vi "Test in Loop.vi"() -> ()   [LabVIEW 2020]
uses:
  99_Reference/LVMQTT-master/Controls/Connection_Return_Codes.ctl
  99_Reference/LVMQTT-master/Controls/QoS.ctl
  99_Reference/LVMQTT-master/Controls/User_Info.ctl
  99_Reference/LVMQTT-master/Controls/Connect_Flags.ctl
  99_Reference/LVMQTT-master/Controls/DUP_Flag.ctl
  99_Reference/LVMQTT-master/Controls/Retain_Flag.ctl
  <vilib>/NI/AMC/Read Termination Message.vi
  <vilib>/NI/AMC/Create Single Message.vi
  <vilib>/NI/AMC/Update Message Routing Info.vi
  <vilib>/NI/AMC/Globals.vi
  <vilib>/NI/AMC/Send Message.vi
  <vilib>/ErrorRing/Error Ring.xnode
  99_Reference/LVMQTT-master/MQTT_Functions.lvlib
  <vilib>/NI/AMC/AMC.lvlib
  <userlib>/_OpenG.lib/time/time.llb/openg_time.lvlib
panel:
  in  "Read":bool
  in  "CMD_0":bool
  in  "Test Connect":bool
  out "Connection Status":T1
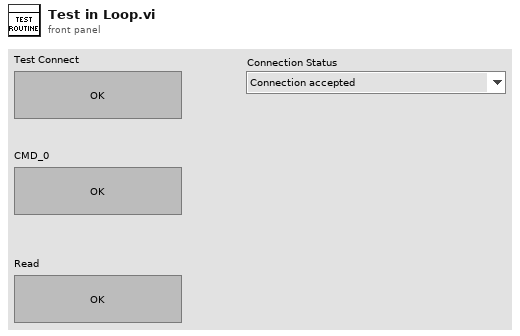
[diagram p1: front panel]
types:
  T1 = typedef "MQTT_Functions.lvlib/Connection_Return_Codes.ctl" = enum16{"Connection accepted", "Connection refused: unacceptable protocol version", "Connection refused: identifier rejected", "Connection refused: Server unavailable", "Connection refused: bad user name or password", "Connection refused: not authorized"}
  T2 = typedef "AMC.lvlib/Message Queue.ctl" = refnum<queue>
  T3 = typedef "MQTT_Functions.lvlib/QoS.ctl" = enum8{"At most once", "At least once", "Exactly once", "Reserved"}
  T4 = typedef "MQTT_Functions.lvlib/Retain_Flag.ctl" = bool
  T5 = typedef "MQTT_Functions.lvlib/DUP_Flag.ctl" = bool
  T6 = cluster{"Hostname":string, "Mac(From)":string, "IP":string, "ConnID":refnum<k5>}
  T7 = cluster{"QoS":T3, "DUP":T5, "Retain":T4, "Keep Alive (sec)":u16}
  T8 = typedef "MQTT_Functions.lvlib/Connect_Flags.ctl" = cluster{"user name":bool, "password":bool, "will retain":bool, "will flag":bool, "clean session":bool, "reserved":bool, "will QoS":T3}
  T9 = typedef "MQTT_Functions.lvlib/User_Info.ctl" = cluster{"User Name":string, "Password":string}
  T10 = cluster{"User Info":T9, "Client ID":string, "MQTT Broker":cluster{"address (IP)":string, "port":u16}, "Connection Status":T1, "Connect Flags":T8, "Connect Meta":cluster{"QoS":T3, "DUP":T5, "Retain":T4, "Keep Alive (sec)":u16}, "MainInfo":cluster{"Hostname":string, "Mac(From)":string, "IP":string, "ConnID":refnum<k5>}, "Channel":string, "tickCount":u32, "tickTarget":u32, "Message ID":u16, "Subscription Info Array":cluster{"Topic":string, "QoS":T3}[]}
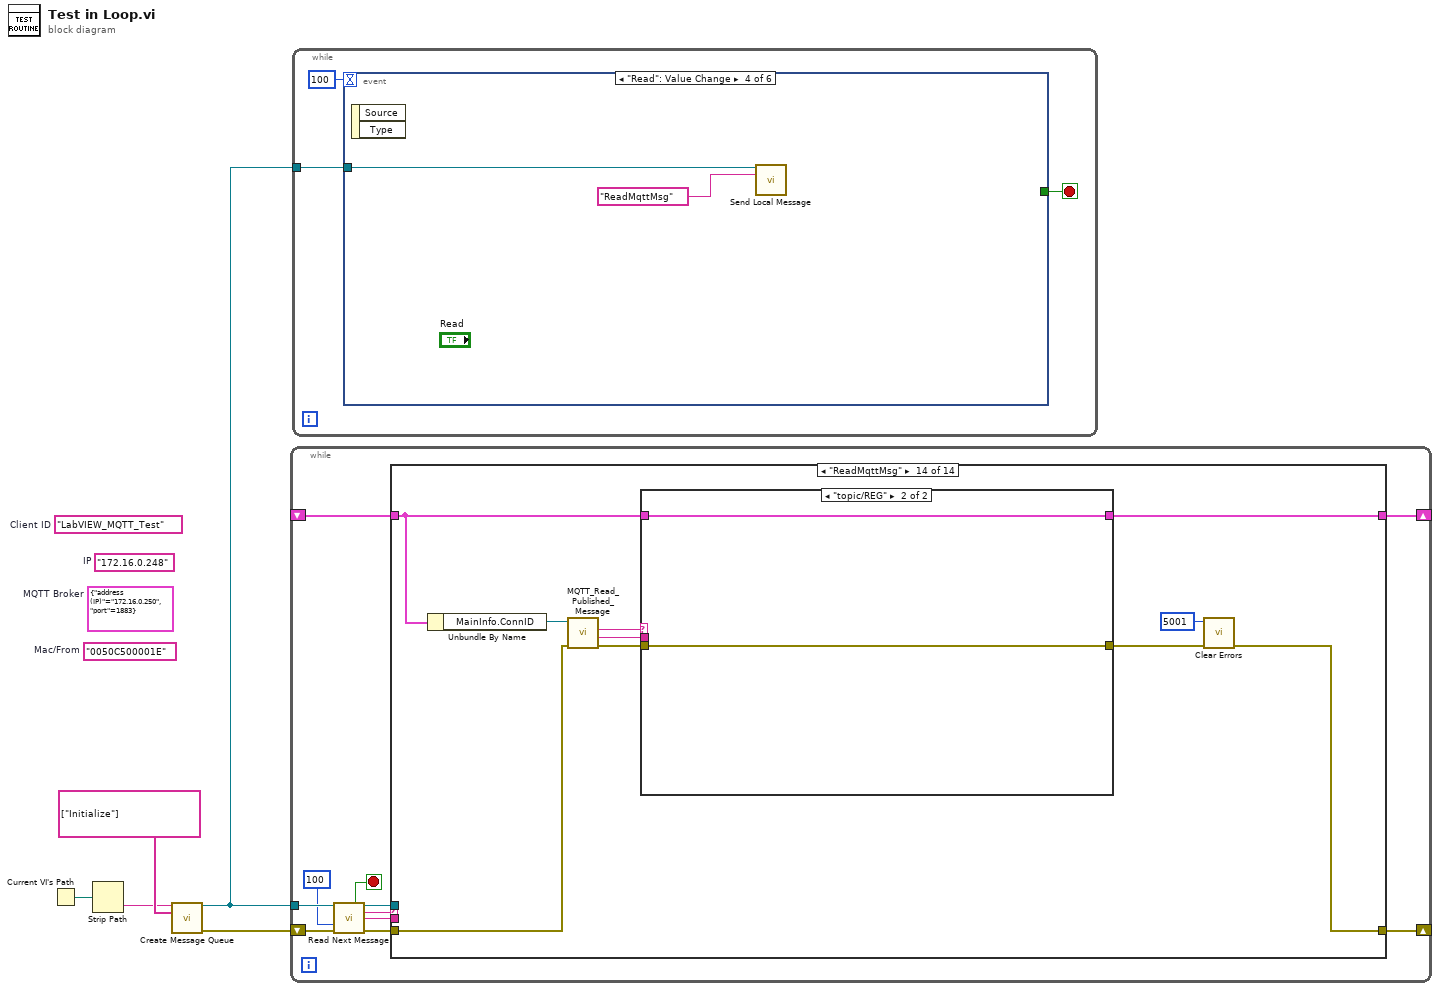
[diagram p0: block diagram]
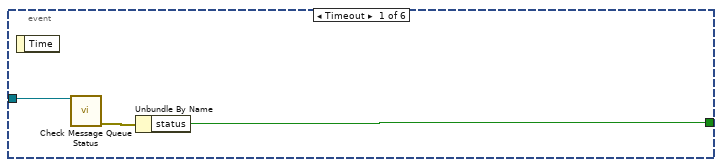
[diagram p2: hidden frame]
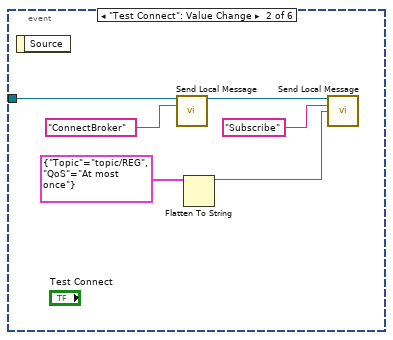
[diagram p3: hidden frame]
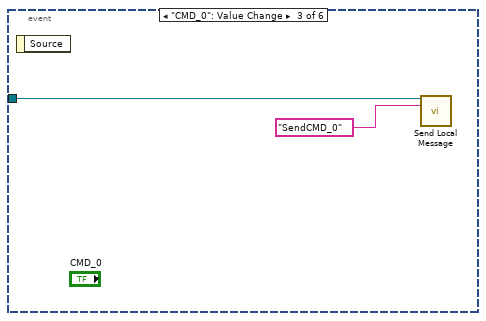
[diagram p4: hidden frame]
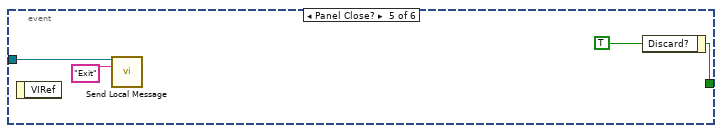
[diagram p5: hidden frame]
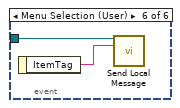
[diagram p6: hidden frame]
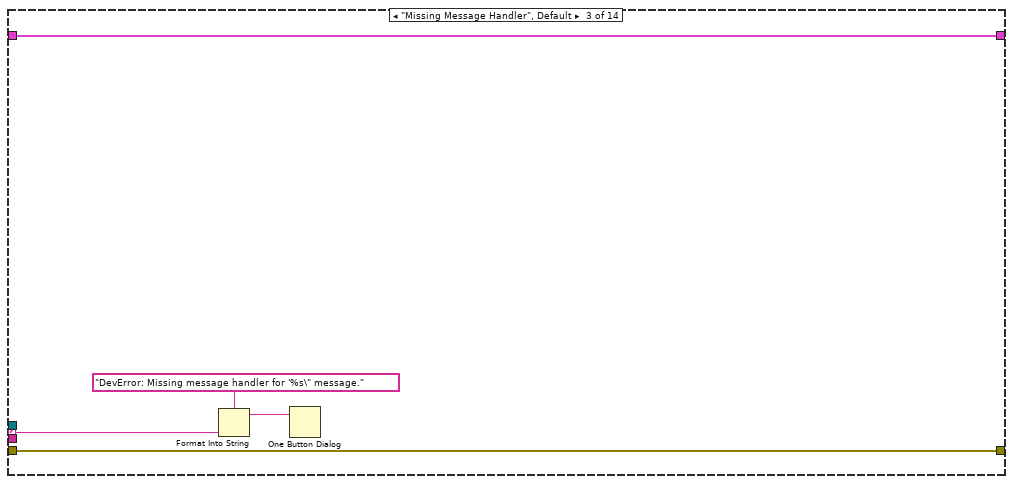
[diagram p9: hidden frame]
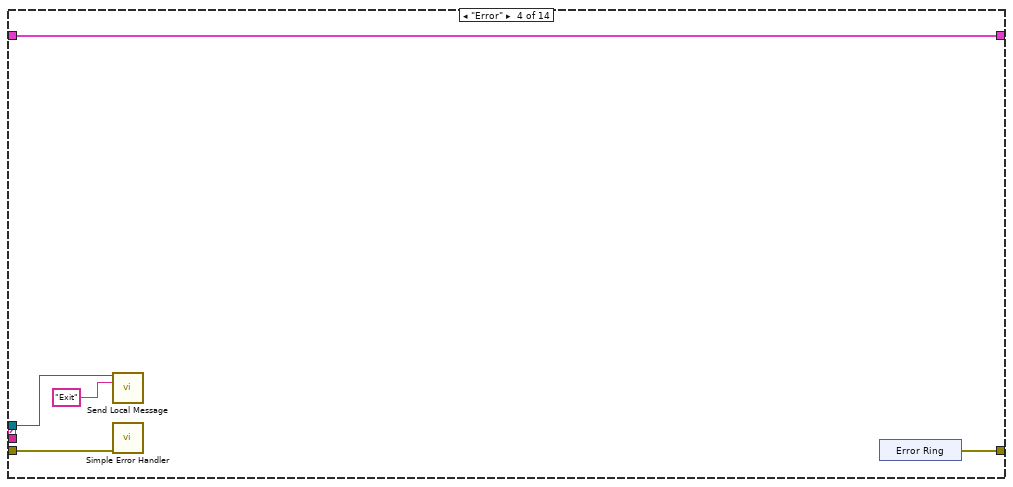
[diagram p10: hidden frame]
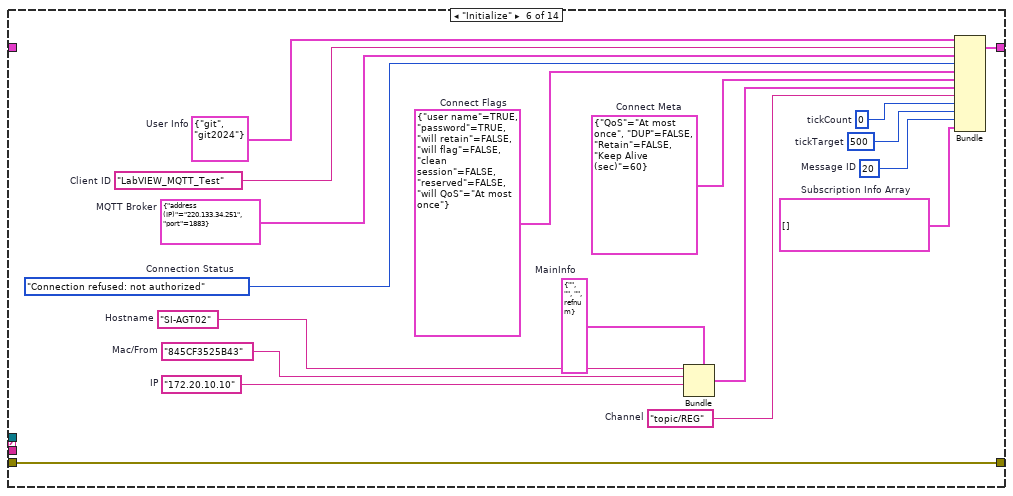
[diagram p12: hidden frame]
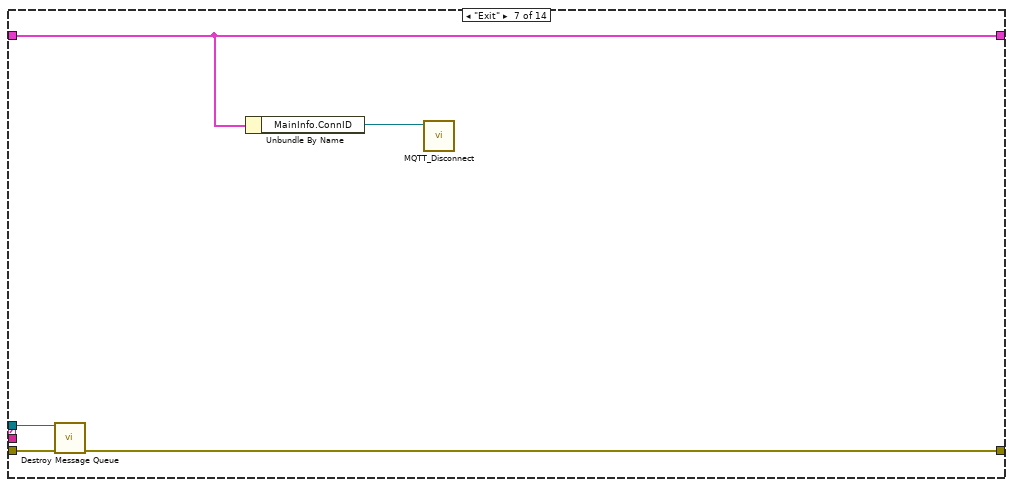
[diagram p13: hidden frame]
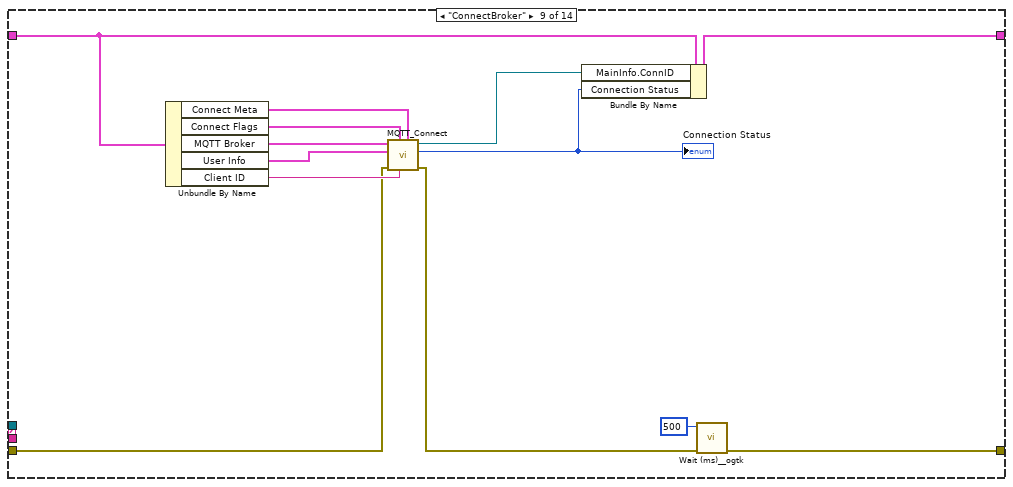
[diagram p15: hidden frame]
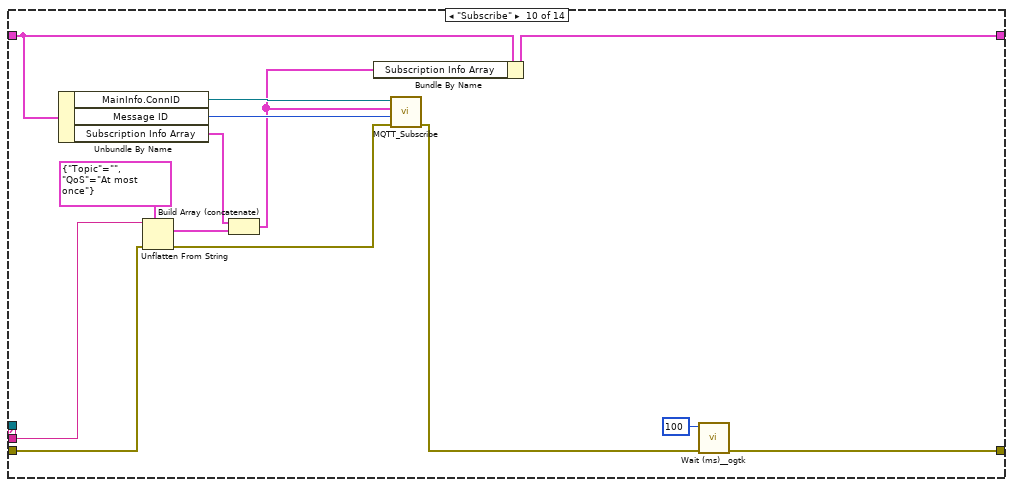
[diagram p16: hidden frame]
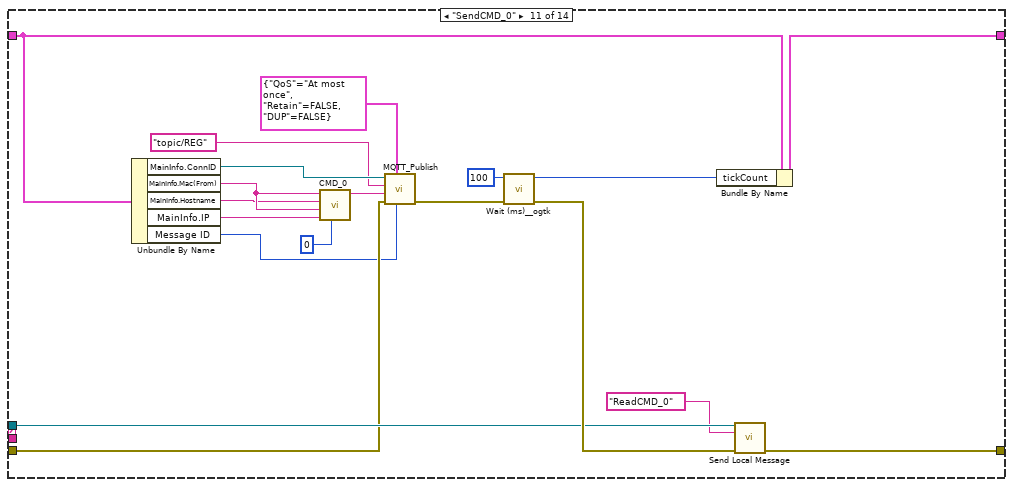
[diagram p17: hidden frame]
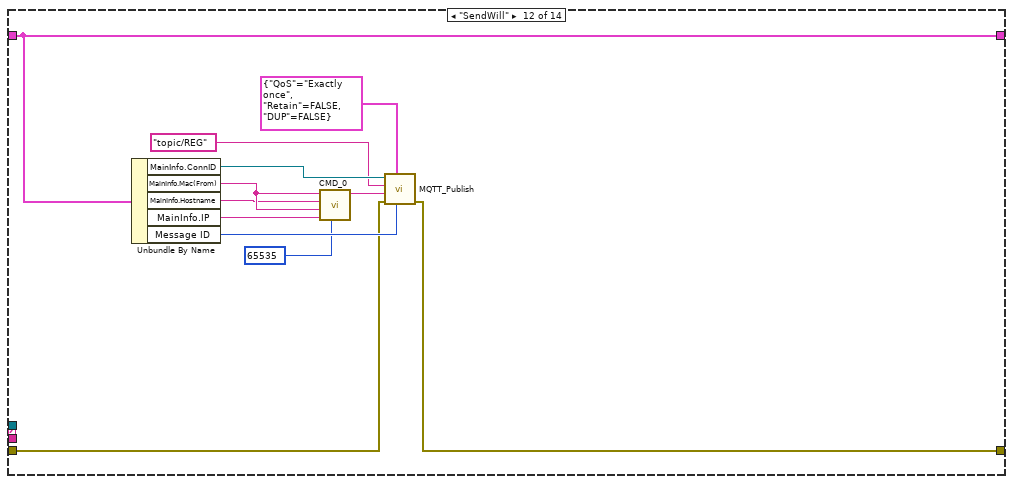
[diagram p18: hidden frame]
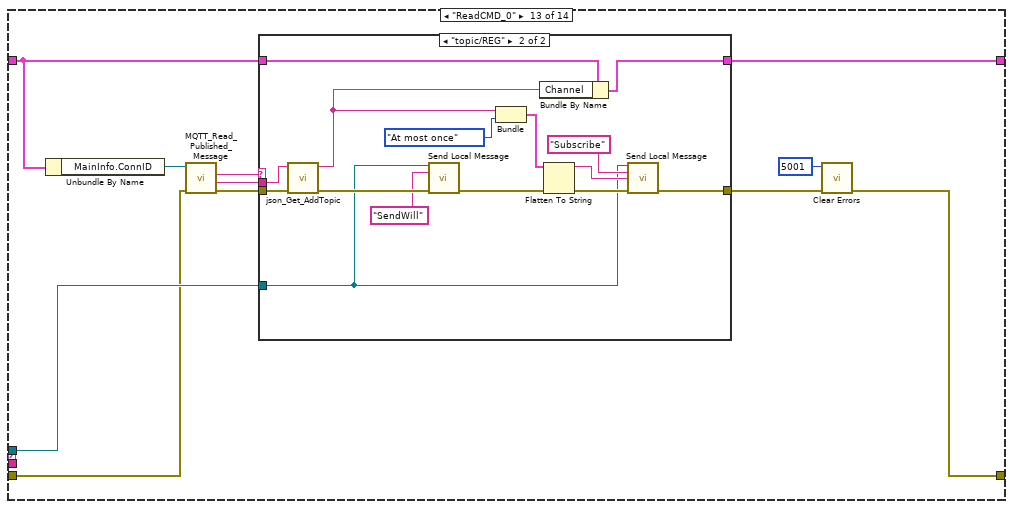
[diagram p19: hidden frame]
diagram:
  (unwired) "LabVIEW_MQTT_Test"  # Client ID
  (unwired) "0050C500001E"  # Mac/From
  (unwired) cluster{"address (IP)":string, "port":u16} {"address (IP)"="172.16.0.250", "port"=1883}  # MQTT Broker
  (unwired) "172.16.0.248"  # IP
  n1 = Current VI's Path() -> (path=w1:path)
  n2 = Strip Path(path=w1) -> (name=w4:string)  [unwired: 1 out]
  n3 = call <vilib>:"Create Message Queue.vi"("message queue name"=w4, "initial message names"=string[] ["Initialize"]) -> ("message queue out"=w3:T2, "error out"=w2:errorcluster)  [unwired: 12 in]
  n4 = while "Message Processor" {
    shift-left: w2 -> [w10]
    shift-right: [w14] -> _
    tunnel: w3 -> [w11]
    shift-left: _ -> [w16]
    shift-right: [w15] -> _
    stop <- w13 stop-if-true
    n5 = call <vilib>:"Read Next Message.vi"("message queue in"=w11, "timeout (1 ms)"=100 ("Timeout"), "error in"=w10) -> ("exit process?"=w13:bool, "message queue out"=w12:T2, "message name"=w8:string, "message value"=w7:string, "error out"=w9:errorcluster)  [unwired: 5 in, 3 out]
    n6 = case shown="\"ReadMqttMsg\"" w8 {
      selector: w8 -> [_ _ w23 _ _ _ _ _ _ _ _ _ _ _]
      tunnel: [w18 w20 w25 w30 w33 w50 w53 w58 w66 w77 w100 w114 w121 w149] -> w15
      tunnel: w16 -> [w18 w20 w25 w30 w33 _ w53 w58 w71 w85 w102 w114 w122 w150]
      tunnel: w12 -> [_ _ _ w29 _ _ w55 _ _ _ w97 _ w123 _]
      tunnel: w9 -> [w17 w19 w24 w27 w32 w51 w56 w57 w61 w74 w90 w107 w119 w147]
      tunnel: [w17 w19 w24 w26 w32 w51 w54 w57 w60 w73 w94 w113 w118 w146] -> w14
      tunnel: w7 -> [_ _ _ _ _ _ _ _ _ w81 _ _ _ _]
      frame "---------- Framework Operations ----------" {
      }
      frame "", "Idle" {
      }
      frame "Missing Message Handler", Default {
        n7 = Format Into String(format string="DevError: Missing message handler for '%s\" message." ("message"), w23) -> (resulting string=w21:string)  [unwired: 2 in, 1 out]
        n8 = One Button Dialog(message=w21) -> ()  [unwired: 2 out]
      }
      frame "Error" {
        n9 = call <vilib>:"Send Local Message.vi"("message queue in"=w29, "message name"="Exit") -> ()  [unwired: 11 in, 3 out]
        n10 = call <vilib>:"Simple Error Handler.vi"("error in (no error)"=w27) -> ()  [unwired: 1 in, 8 out]
        n11 = xnode "Error Ring"() -> ("error out"=w26:errorcluster)
      }
      frame "---------- Generic Operations ----------" {
      }
      frame "Initialize" {
        w34 = cluster{"Topic":string, "QoS":T3}[] []  # Subscription Info Array
        w35 = u16 20  # Message ID
        w36 = u32 500  # tickTarget
        w37 = u32 0  # tickCount
        w38 = "topic/REG"  # Channel
        w39 = T6 {"Hostname"="", "Mac(From)"="", "IP"="", "ConnID"=refnum}  # MainInfo
        w42 = "845CF3525B43"  # Mac/From
        w41 = "SI-AGT02"  # Hostname
        w43 = "172.20.10.10"  # IP
        w44 = T7 {"QoS"=enum."At most once", "DUP"=FALSE, "Retain"=FALSE, "Keep Alive (sec)"=60}  # Connect Meta
        w45 = T8 {"user name"=TRUE, "password"=TRUE, "will retain"=FALSE, "will flag"=FALSE, "clean session"=FALSE, "reserved"=FALSE, "will QoS"=enum."At most once"}  # Connect Flags
        w46 = Connection_Return_Codes."Connection refused: not authorized"  # Connection Status
        w47 = cluster{"address (IP)":string, "port":u16} {"address (IP)"="220.133.34.251", "port"=1883}  # MQTT Broker
        w48 = "LabVIEW_MQTT_Test"  # Client ID
        w49 = T9 {"User Name"="git", "Password"="git2024"}  # User Info
        n12 = Bundle(cluster=w39, "Hostname"=w41, "Mac(From)"=w42, "IP"=w43) -> (w40:T6)  [unwired: 1 in]
        n13 = Bundle("User Info"=w49, "Client ID"=w48, "MQTT Broker"=w47, "Connection Status"=w46, "Connect Flags"=w45, "Connect Meta"=w44, "MainInfo"=w40, "Channel"=w38, "tickCount"=w37, "tickTarget"=w36, "Message ID"=w35, "Subscription Info Array"=w34) -> (w50:T10)  [unwired: 1 in]
      }
      frame "Exit" {
        n14 = call <vilib>:"Destroy Message Queue.vi"("message queue in"=w55, "error in"=w56) -> ("error out"=w54:errorcluster)  [unwired: 11 in, 2 out]
        n15 = Unbundle By Name(w53) -> ("MainInfo.ConnID"=w52:refnum<k5>)
        n16 = call "MQTT_Disconnect.vi"("connection ID"=w52) -> ()  [unwired: 10 in, 1 out]
      }
      frame "---------- Application Operations ----------" {
        # "Dummy case to add a seperator in the Case Structure menu"
      }
      frame "ConnectBroker" {
        n17 = Unbundle By Name(w71) -> ("Connect Meta"=w64:T7, "Connect Flags"=w63:T8, "MQTT Broker"=w70:cluster{"address (IP)":string, "port":u16}, "User Info"=w69:T9, "Client ID"=w68:string)
        n18 = call "MQTT_Connect.vi"("Connect Meta"=w64, "Client ID"=w68, "Connect Flags"=w63, "error in (no error)"=w61, "User Info"=w69, "MQTT Broker"=w70) -> ("error out"=w67:errorcluster, "Connection Status"=w65:T1, "connection ID out"=w62:refnum<k5>)  [unwired: 3 in]
        "Connection Status" <- w65
        n19 = Bundle By Name(cluster=w71, "MainInfo.ConnID"=w62, "Connection Status"=w65) -> (w66:T10)
        n20 = call <userlib>:"Wait (ms)__ogtk.vi"("error in (no error)"=w67, "milliseconds to wait"=u32 500) -> ("error out"=w60:errorcluster)  [unwired: 8 in, 1 out]
      }
      frame "Subscribe" {
        n21 = Unbundle By Name(w85) -> ("MainInfo.ConnID"=w84:refnum<k5>, "Message ID"=w82:u16, "Subscription Info Array"=w79:cluster{"Topic":string, "QoS":T3}[])
        n22 = Unflatten From String(type=cluster{"Topic":string, "QoS":T3} {"Topic"="", "QoS"=enum."At most once"} ("Subscription Info"), binary string=w81, error in (no error)=w74) -> (value=w78:cluster{"Topic":string, "QoS":T3}, error out=w75:errorcluster)  [unwired: 2 in, 1 out]
        n23 = Build Array (concatenate)(w79, w78) -> (w76:cluster{"Topic":string, "QoS":T3}[])
        n24 = Bundle By Name(cluster=w85, "Subscription Info Array"=w76) -> (w77:T10)
        n25 = call "MQTT_Subscribe.vi"("error in (no error)"=w75, "Message ID"=w82, "Subscription Info Array"=w76, "connection ID"=w84) -> ("error out"=w83:errorcluster)  [unwired: 6 in, 1 out]
        n26 = call <userlib>:"Wait (ms)__ogtk.vi"("error in (no error)"=w83, "milliseconds to wait"=u32 100) -> ("error out"=w73:errorcluster)  [unwired: 8 in, 1 out]
      }
      frame "SendCMD_0" {
        n27 = Unbundle By Name(w102) -> ("MainInfo.ConnID"=w104:refnum<k5>, "MainInfo.Mac(From)"=w92:string, "MainInfo.Hostname"=w91:string, "MainInfo.IP"=w93:string, "Message ID"=w86:u16)
        n28 = call "CMD_0.vi"("CMD"=u32 0, "IP"=w93, "MAC"=w92, "HOSTNAME"=w91, "Mac/From"=w92) -> ("JSON String"=w103:string)  [unwired: 6 in]
        n29 = call "MQTT_Publish.vi"("Message ID"=w86, "Publish Meta"=cluster{"QoS":T3, "Retain":T4, "DUP":T5} {"QoS"=enum."At most once", "Retain"=FALSE, "DUP"=FALSE}, "error in (no error)"=w90, "Message to be published"=w103, "Topic"="topic/REG", "connection ID"=w104) -> ("error out"=w101:errorcluster)  [unwired: 4 in, 1 out]
        n30 = call <userlib>:"Wait (ms)__ogtk.vi"("error in (no error)"=w101, "milliseconds to wait"=u32 100) -> ("error out"=w98:errorcluster, "millisecond timer value"=w99:u32)  [unwired: 8 in]
        n31 = Bundle By Name(cluster=w102, "tickCount"=w99) -> (w100:T10)
        n32 = call <vilib>:"Send Local Message.vi"("message queue in"=w97, "message name"="ReadCMD_0", "error in"=w98) -> ("error out"=w94:errorcluster)  [unwired: 10 in, 2 out]
      }
      frame "SendWill" {
        n33 = Unbundle By Name(w114) -> ("MainInfo.ConnID"=w116:refnum<k5>, "MainInfo.Mac(From)"=w110:string, "MainInfo.Hostname"=w109:string, "MainInfo.IP"=w111:string, "Message ID"=w108:u16)
        n34 = call "CMD_0.vi"("CMD"=u32 65535, "IP"=w111, "MAC"=w110, "HOSTNAME"=w109, "Mac/From"=w110) -> ("JSON String"=w115:string)  [unwired: 6 in]
        n35 = call "MQTT_Publish.vi"("Message ID"=w108, "Publish Meta"=cluster{"QoS":T3, "Retain":T4, "DUP":T5} {"QoS"=enum."Exactly once", "Retain"=FALSE, "DUP"=FALSE}, "error in (no error)"=w107, "Message to be published"=w115, "Topic"="topic/REG", "connection ID"=w116) -> ("error out"=w113:errorcluster)  [unwired: 4 in, 1 out]
      }
      frame "ReadCMD_0" {
        n36 = Unbundle By Name(w122) -> ("MainInfo.ConnID"=w127:refnum<k5>)
        n37 = call "MQTT_Read_Published_Message.vi"("error in (no error)"=w119, "connection ID"=w127) -> ("error out"=w124:errorcluster, "Message"=w125:string, "Topic Name"=w126:string)  [unwired: 4 in, 3 out]
        n38 = case shown="\"topic/REG\"" w126 {
          tunnel: w125 -> [_ w144]
          tunnel: w124 -> [w128 w143]
          tunnel: w123 -> [_ w131]
          tunnel: w122 -> [w129 w137]
          tunnel: [w129 w136] -> w121
          tunnel: [w128 w130] -> w120
          frame "False", Default {
          }
          frame "topic/REG" {
            n39 = call "json_Get_AddTopic.vi"("error in"=w143, "ReadCMD_0"=w144) -> ("error out"=w133:errorcluster, "AddTopic"=w135:string)  [unwired: 8 in]
            n40 = call <vilib>:"Send Local Message.vi"("message queue in"=w131, "message name"="SendWill", "error in"=w133) -> ("error out"=w134:errorcluster)  [unwired: 10 in, 2 out]
            n41 = Bundle("AddTopic"=w135, "QoS"=QoS."At most once") -> (w140:cluster{"AddTopic":string, "QoS":T3})  [unwired: 1 in]
            n42 = Bundle By Name(cluster=w137, "Channel"=w135) -> (w136:T10)
            n43 = Flatten To String(anything=w140, error in (no error)=w134) -> (data string=w139:string, error out=w138:errorcluster)  [unwired: 2 in, 1 out]
            n44 = call <vilib>:"Send Local Message.vi"("message queue in"=w131, "message name"="Subscribe", "message value"=w139, "error in"=w138) -> ("error out"=w130:errorcluster)  [unwired: 9 in, 2 out]
          }
        }
        n45 = call <vilib>:"Clear Errors.vi"("error in (no error)"=w120, "specific error code to clear (0: all)"=5001) -> ("error out"=w118:errorcluster)  [unwired: 4 in, 1 out]
      }
      frame "ReadMqttMsg" {
        n46 = Unbundle By Name(w150) -> ("MainInfo.ConnID"=w154:refnum<k5>)
        n47 = call "MQTT_Read_Published_Message.vi"("error in (no error)"=w147, "connection ID"=w154) -> ("error out"=w151:errorcluster, "Message"=w152:string, "Topic Name"=w153:string)  [unwired: 4 in, 3 out]
        n48 = case shown="\"topic/REG\"" w153 {
          tunnel: w152 -> [_ _]
          tunnel: w151 -> [w155 w157]
          tunnel: w150 -> [w156 w158]
          tunnel: [w156 w158] -> w149
          tunnel: [w155 w157] -> w148
          frame "False", Default {
          }
          frame "topic/REG" {
          }
        }
        n49 = call <vilib>:"Clear Errors.vi"("error in (no error)"=w148, "specific error code to clear (0: all)"=5001) -> ("error out"=w146:errorcluster)  [unwired: 4 in, 1 out]
      }
    }
  }
  n50 = while "Message Generator - User Interface Event Handler" {
    tunnel: w3 -> [w159]
    stop <- w160 stop-if-true
    n51 = event shown="[3] \"Read\": Value Change" {
      selector: _ -> [_ _ _ _ _ _]
      dyn-events: _ -> [_ _ _ _ _ _]
      timeout: 100 ("Event Structure Timeout (ms)") -> [_ _ _ _ _ _]
      tunnel: [w162 _ _ _ w177 _] -> w160
      tunnel: w159 -> [w163 w170 w172 w174 w175 w178]
      event Timeout {
        n52 = event-data() -> ()  [unwired: 2 out]
        n53 = call <vilib>:"Check Message Queue Status.vi"("message queue in"=w163) -> ("error out"=w164:errorcluster)  [unwired: 10 in, 4 out]
        n54 = Unbundle By Name(w164) -> ("status"=w162:bool)
      }
      event "Test Connect": Value Change {
        n55 = event-data() -> ()  [unwired: 2 out]
        n56 = call <vilib>:"Send Local Message.vi"("message queue in"=w170, "message name"="ConnectBroker") -> ("message queue out"=w167:T2)  [unwired: 11 in, 2 out]
        n57 = Flatten To String(anything=cluster{"Topic":string, "QoS":T3} {"Topic"="topic/REG", "QoS"=enum."At most once"} ("Subscription Info")) -> (data string=w165:string)  [unwired: 3 in, 2 out]
        n58 = call <vilib>:"Send Local Message.vi"("message queue in"=w167, "message name"="Subscribe", "message value"=w165) -> ()  [unwired: 10 in, 3 out]
      }
      event "CMD_0": Value Change {
        n59 = event-data() -> ()  [unwired: 2 out]
        n60 = call <vilib>:"Send Local Message.vi"("message queue in"=w172, "message name"="SendCMD_0") -> ()  [unwired: 11 in, 3 out]
      }
      event "Read": Value Change {
        n61 = event-data() -> ()  [unwired: 3 out]
        n62 = call <vilib>:"Send Local Message.vi"("message queue in"=w174, "message name"="ReadMqttMsg") -> ()  [unwired: 11 in, 3 out]
      }
      event Panel Close? {
        w177 = TRUE ("Discard?")
        n63 = event-data() -> ()  [unwired: 2 out]
        n64 = call <vilib>:"Send Local Message.vi"("message queue in"=w175, "message name"="Exit") -> ()  [unwired: 11 in, 3 out]
        n65 = event-data("Discard?"=w177) -> ()  [unwired: 1 in, 1 out]
      }
      event Menu Selection (User) {
        n66 = event-data() -> ("ItemTag"=w179:string)  [unwired: 1 out]
        n67 = call <vilib>:"Send Local Message.vi"("message queue in"=w178, "message name"=w179) -> ()  [unwired: 11 in, 3 out]
      }
    }
  }
